vi "Convert Missing Parameters into Error.vi"(6 "Parameter":variant, 8 "Missing Parameters in":errorcluster) -> (0 "Missing Parameters out":errorcluster)   [LabVIEW 2023, in "Request.lvclass"]
doc: "Helper SubVI that sets an error when the Request is missing parameters. (Used when an Endpoint/Request needs parameters.)"
uses:
  Request.lvclass
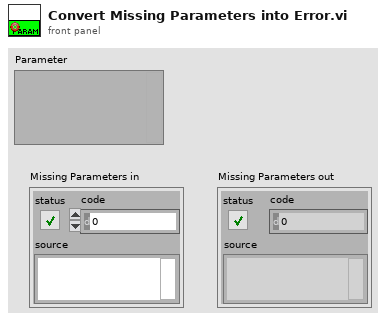
[diagram p1: front panel]
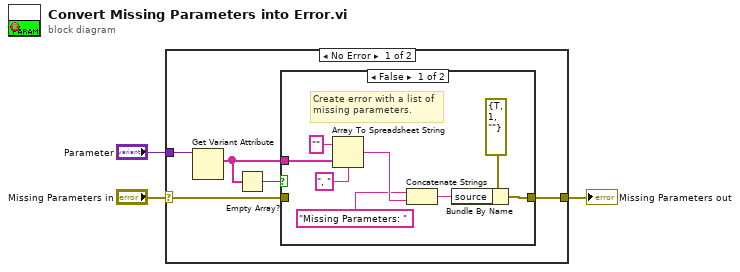
[diagram p0: block diagram]
diagram:
  n1 = case shown="No Error" "Missing Parameters in" {
    selector: "Missing Parameters in" -> [w6 w18]
    tunnel: [w5 w18] -> w2
    tunnel: "Parameter" -> [w8 _]
    frame No Error {
      n2 = Get Variant Attribute(Variant=w8) -> (names=w4:string[])  [unwired: 3 in, 3 out]
      n3 = Empty Array?(array=w4) -> (empty?=w7:bool)
      n4 = case shown="False" w7 {
        tunnel: w6 -> [_ w17]
        tunnel: [w16 w17] -> w5
        tunnel: w4 -> [w14 _]
        frame False {
          # "Create error with a list of\nmissing parameters."
          n5 = Array To Spreadsheet String(delimiter (Tab)=", ", array=w14, 3:"" ("format string")) -> (spreadsheet string=w10:string)
          n6 = Concatenate Strings("Missing Parameters: " ("format string"), w10) -> (w11:string)
          n7 = Bundle By Name(cluster=errorcluster {"status"=TRUE, "code"=1, "source"=""} ("error IO"), "source"=w11) -> (w16:errorcluster)
        }
        frame True {
          # "No missing parameters, do not create\nerror."
        }
      }
    }
    frame Error {
    }
  }
  "Missing Parameters out" <- w2
